vi "Gestore Cluster valvole.vi"(6 "Enum":enum16{"Inizializza cluster", "Set value"}(ring)=enum."Set value", 8 "Cluster INFO":T1={"Scelta wattmetro"={"Wattmetro"=enum."No Selection"}, "SET RPM"=0.0, "SET TEMP"=0.0, "Costanti collaudo"={"P [bar]"=0.0, "T amb. [°C]"=0.0, "Umidità [%]"=0.0, "T acqua [°C] 2"=0.0}, "Array linee"=[{"portata"=0, "Hasp"=0, "Hmand"=1, "Torsiometro"=0, "rpm"=0, "Hdiff?"=FALSE, "T amb"=0, "Indici valvole"=[0, 1], "Nome"="Elettropompa", "Sommersa?"=FALSE, "nomi valvole"=[]}, {"portata"=1, "Hasp"=0, "Hmand"=0, "Torsiometro"=0, "rpm"=0, "Hdiff?"=FALSE, "T amb"=0, "Indici valvole"=[0, 1], "Nome"="Sommersa", "Sommersa?"=TRUE, "nomi valvole"=[]}], "Array valvole linee avvio/fermata"=[], "Linea selezionata"=0.0, "Sett T e R"={"Tamb[°C]"=0.0, "Ru-w"=0.0, "Rmarcia"=0.0, "Raux"=0.0, "Tamb Freddo[°C]"=0.0, "Ru-w freddo"=0.0, "Rmarcia freddo"=0.0, "Raux freddop"=0.0, "TC1"=0.0, "TC2"=0.0, "TC3"=0.0, "TC4"=0.0, "TC5"=0.0, "TC6"=0.0, "TC7"=0.0, "TC8"=0.0}, "Nomi valvole prop sistema"=[], "mandata"={"canale"="", "ai min"=0.0, "ai max"=0.0, "range"=0.0, "offset"=0.0, "UM"=enum."V"}, "aspirazione"={"canale"="", "ai min"=0.0, "ai max"=0.0, "range"=0.0, "offset"=0.0, "UM"=enum."V"}, "Array portate"=[], "canale-- sensore"=[], "Premistoppa"={"canale"="", "ai min"=0.0, "ai max"=0.0, "range"=0.0, "offset"=0.0, "UM"=enum."V"}, "Coppia"={"canale"="", "ai min"=0.0, "ai max"=0.0, "range"=0.0, "offset"=0.0, "UM"=enum."V"}, "Attriti B1"=[], "Attriti B2"=[], "Collegamento elettrico"={"ALIMENTAZIONE ELETTRICA"=enum."AC TRIFASE", "ID"=0.0}}, 10 "stato valvole sistema":dbl[](array[numeric]), 11 "Cluster valvole":refnum<vi>) -> ()   [LabVIEW 2016]
uses:
  TypeDef/Cluster INFO.ctl
  TypeDef/WT SELECTION.ctl
  TypeDef/Definizione linea.ctl
  TypeDef/sett T e R.ctl
  TypeDef/Collegamenti_elettrici.ctl
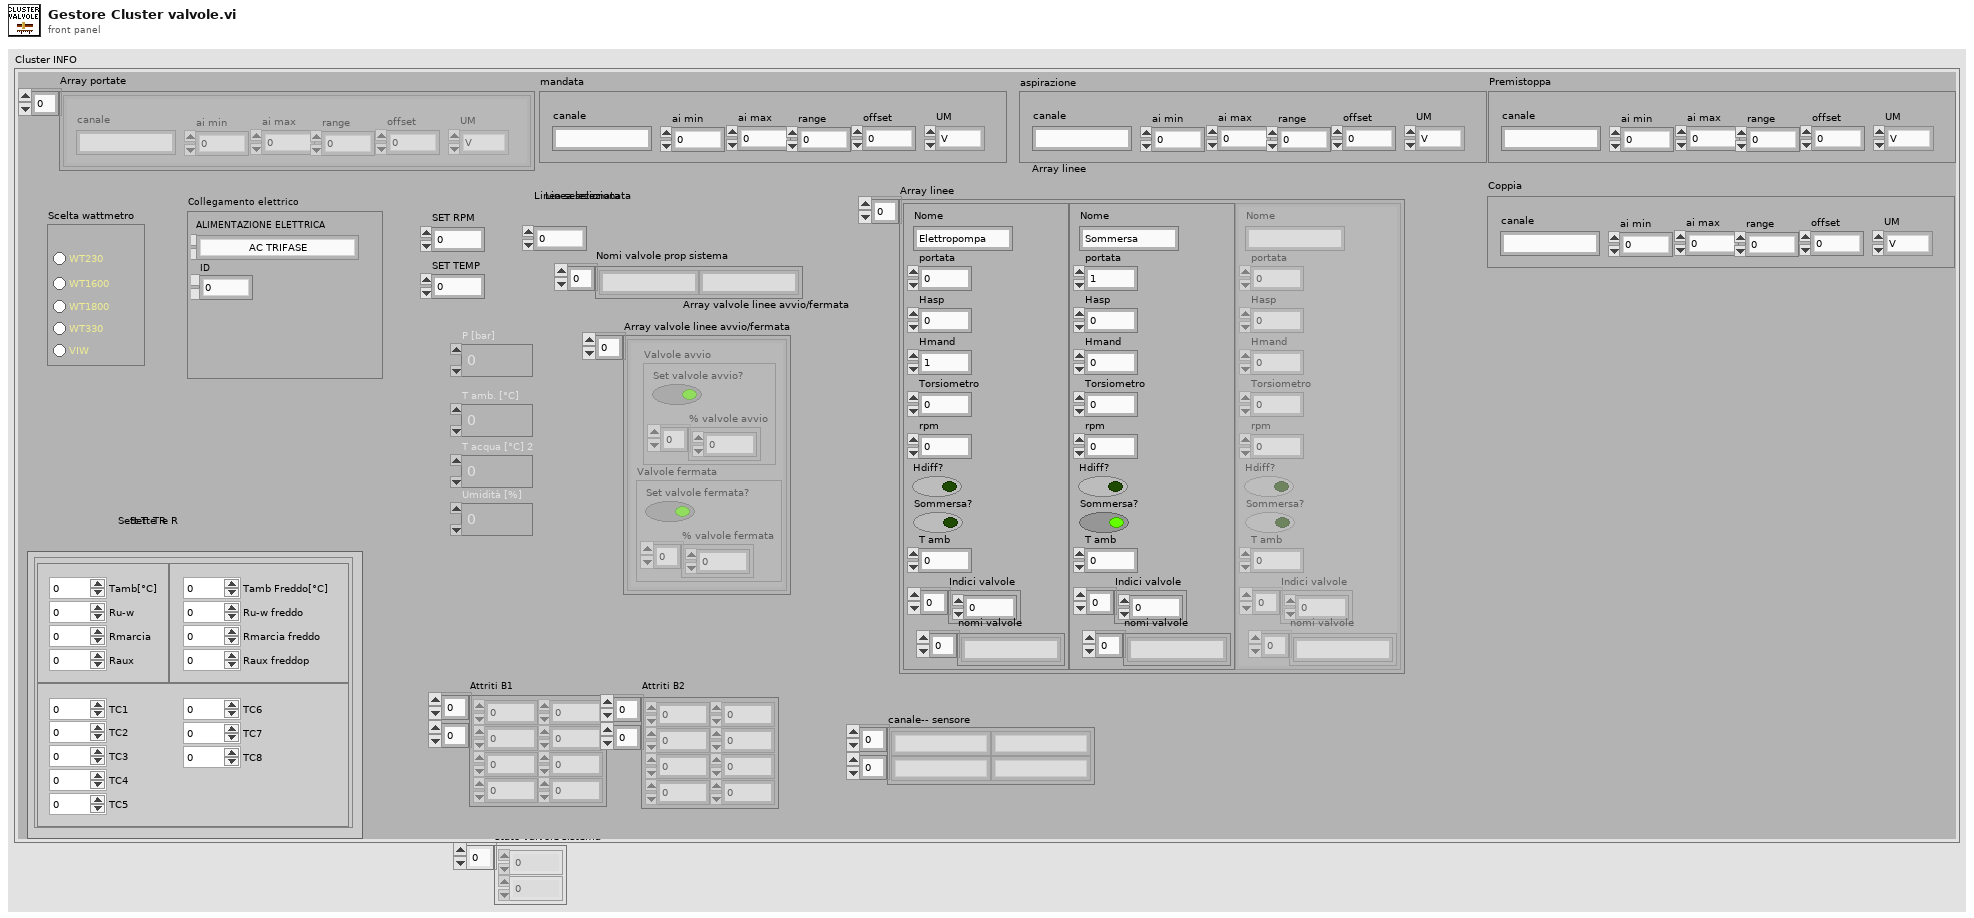
[diagram p1: front panel]
types:
  T1 = typedef "Cluster INFO.ctl" = cluster{"Scelta wattmetro":cluster{"Wattmetro":T2}, "SET RPM":dbl, "SET TEMP":dbl, "Costanti collaudo":cluster{"P [bar]":dbl, "T amb. [°C]":dbl, "Umidità [%]":dbl, "T acqua [°C] 2":dbl}, "Array linee":T3[], "Array valvole linee avvio/fermata":cluster{"Valvole avvio":cluster{"Set valvole avvio?":bool, "% valvole avvio":dbl[]}, "Valvole fermata":cluster{"Set valvole fermata?":bool, "% valvole fermata":dbl[]}}[], "Linea selezionata":dbl, "Sett T e R":T4, "Nomi valvole prop sistema":string[], "mandata":cluster{"canale":string, "ai min":dbl, "ai max":dbl, "range":dbl, "offset":dbl, "UM":T5}, "aspirazione":cluster{"canale":string, "ai min":dbl, "ai max":dbl, "range":dbl, "offset":dbl, "UM":T5}, "Array portate":cluster{"canale":string, "ai min":dbl, "ai max":dbl, "range":dbl, "offset":dbl, "UM":T5}[], "canale-- sensore":string[][], "Premistoppa":cluster{"canale":string, "ai min":dbl, "ai max":dbl, "range":dbl, "offset":dbl, "UM":T5}, "Coppia":cluster{"canale":string, "ai min":dbl, "ai max":dbl, "range":dbl, "offset":dbl, "UM":T5}, "Attriti B1":dbl[][], "Attriti B2":dbl[][], "Collegamento elettrico":cluster{"ALIMENTAZIONE ELETTRICA":T6, "ID":dbl}}
  T2 = typedef "WT SELECTION.ctl" = enum32{"No Selection", "WT230", "WT1600", "WT1800", "WT330", "VIW"}
  T3 = typedef "Definizione linea.ctl" = cluster{"portata":i32, "Hasp":i32, "Hmand":i32, "Torsiometro":i32, "rpm":i32, "Hdiff?":bool, "T amb":i32, "Indici valvole":i16[], "Nome":string, "Sommersa?":bool, "nomi valvole":string[]}
  T4 = typedef "sett T e R.ctl" = cluster{"Tamb[°C]":dbl, "Ru-w":dbl, "Rmarcia":dbl, "Raux":dbl, "Tamb Freddo[°C]":dbl, "Ru-w freddo":dbl, "Rmarcia freddo":dbl, "Raux freddop":dbl, "TC1":dbl, "TC2":dbl, "TC3":dbl, "TC4":dbl, "TC5":dbl, "TC6":dbl, "TC7":dbl, "TC8":dbl}
  T5 = typedef "UnitàMisura.ctl" = enum16{"V", "mA", "Bar", "RPM", "m3/s", "m3/min", "m3/h", "l/s", "l/min", "in3/min", "ft3/min", "gpm", "igpm", "igph", "%", "°C", "m", "Nm"}
  T6 = typedef "Collegamenti_elettrici.ctl" = enum16{"AC TRIFASE", "AC MONOFASE", "DC CON ECCITAZIONE", "DC NO ECCITAZIONE", "SCORTA 1", "SCORTA 2"}
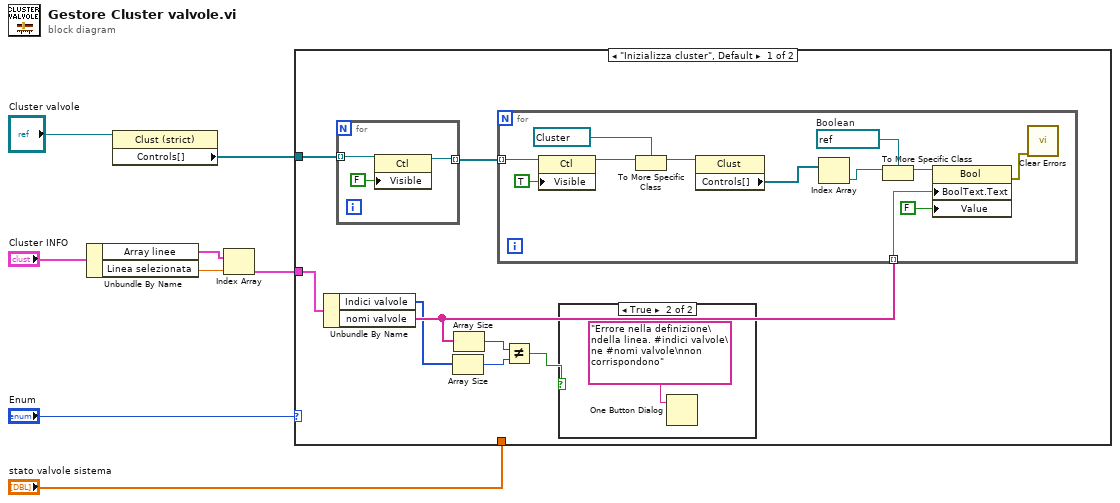
[diagram p0: block diagram]
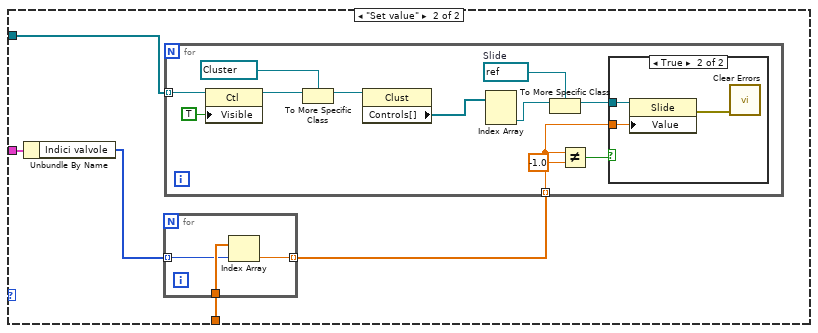
[diagram p3: hidden frame]
diagram:
  n1 = Unbundle By Name("Cluster INFO") -> ("Array linee"=w2:T3[], "Linea selezionata"=w1:dbl)
  n2 = property class="Clust (strict)"(reference="Cluster valvole") -> ("Controls[]"=w8:refnum<vi>[])  [unwired: 1 in, 2 out]
  n3 = Index Array(array=w2, index=w1) -> (element=w5:T3)
  n4 = case shown="\"Inizializza cluster\", Default" "Enum" {
    tunnel: w8 -> [w16 w37]
    tunnel: w5 -> [w14 w36]
    tunnel: "stato valvole sistema" -> [_ w35]
    frame "Inizializza cluster", Default {
      n5 = Unbundle By Name(w14) -> ("Indici valvole"=w12:i16[], "nomi valvole"=w13:string[])
      n6 = for {
        tunnel: w16 -> [w32] mode=indexing
        tunnel: [w30] -> w15 mode=indexing
        n7 = property class="Ctl"(reference=w32, "Visible"=FALSE) -> (reference out=w30:refnum<vi>)  [unwired: 1 in, 1 out]
      }
      n8 = Array Size(array=w12) -> (size(s)=w11:i32)
      n9 = Array Size(array=w13) -> (size(s)=w10:i32)
      n10 = for {
        tunnel: w15 -> [w29] mode=indexing
        tunnel: w13 -> [w23] mode=indexing
        w22 = refnum<vi> refnum  # Boolean
        n11 = property class="Ctl"(reference=w29, "Visible"=TRUE) -> (reference out=w27:refnum<vi>)  [unwired: 1 in, 1 out]
        n12 = To More Specific Class(target class=refnum<vi> refnum ("Valvola 3"), reference=w27) -> (specific class reference=w25:refnum<vi>)  [unwired: 1 in, 1 out]
        n13 = property class="Clust"(reference=w25) -> ("Controls[]"=w21:refnum<vi>[])  [unwired: 1 in, 2 out]
        n14 = Index Array(array=w21) -> (element=w20:refnum<vi>)  [unwired: 1 in]
        n15 = To More Specific Class(target class=w22, reference=w20) -> (specific class reference=w24:refnum<vi>)  [unwired: 1 in, 1 out]
        n16 = property class="Bool"(reference=w24, "BoolText.Text"=w23, "Value"=FALSE) -> (error out=w19:errorcluster)  [unwired: 1 in, 1 out]
        n17 = call <vilib>:"Clear Errors.vi"("error in (no error)"=w19) -> ()  [unwired: 5 in, 2 out]
      }
      n18 = Not Equal?(x=w10, y=w11) -> (x != y?=w9:bool)
      n19 = case shown="True" w9 {
        frame False {
        }
        frame True {
          n20 = One Button Dialog(message="Errore nella definizione\ndella linea. #indici valvole\ne #nomi valvole\nnon corrispondono") -> ()  [unwired: 1 in, 1 out]
        }
      }
    }
    frame "Set value" {
      n21 = Unbundle By Name(w36) -> ("Indici valvole"=w34:i16[])
      n22 = for {
        tunnel: w35 -> [w40]
        tunnel: w34 -> [w39] mode=indexing
        tunnel: [w38] -> w33 mode=indexing
        n23 = Index Array(array=w40, index=w39) -> (element=w38:dbl)
      }
      n24 = for {
        tunnel: w37 -> [w52] mode=indexing
        tunnel: w33 -> [w43] mode=indexing
        w46 = refnum<vi> refnum  # Slide
        n25 = property class="Ctl"(reference=w52, "Visible"=TRUE) -> (reference out=w50:refnum<vi>)  [unwired: 1 in, 1 out]
        n26 = To More Specific Class(target class=refnum<vi> refnum ("Valvola 3"), reference=w50) -> (specific class reference=w48:refnum<vi>)  [unwired: 1 in, 1 out]
        n27 = property class="Clust"(reference=w48) -> ("Controls[]"=w45:refnum<vi>[])  [unwired: 1 in, 2 out]
        n28 = Index Array(array=w45) -> (element #2=w44:refnum<vi>)  [unwired: 2 in, 1 out]
        n29 = To More Specific Class(target class=w46, reference=w44) -> (specific class reference=w47:refnum<vi>)  [unwired: 1 in, 1 out]
        n30 = Not Equal?(x=w43, y=-1.0) -> (x != y?=w41:bool)
        n31 = case shown="True" w41 {
          tunnel: w47 -> [_ w55]
          tunnel: w43 -> [_ w53]
          frame False {
          }
          frame True {
            n32 = property class="Slide"(reference=w55, "Value"=w53) -> (error out=w54:errorcluster)  [unwired: 1 in, 1 out]
            n33 = call <vilib>:"Clear Errors.vi"("error in (no error)"=w54) -> ()  [unwired: 5 in, 2 out]
          }
        }
      }
    }
  }
